vi "Read_Parse.vi"(0 "string in":string, 3 "Cluster in":T3) -> (1 "All Data":string, 4 "Motor DataString":string, 5 "DADES":T2, 6 "Acceleròmetre":T1, 7 "Giroscopi":T1, 9 "Magnetometre":T1, 10 "Cluster out":T3)   [LabVIEW 2018]
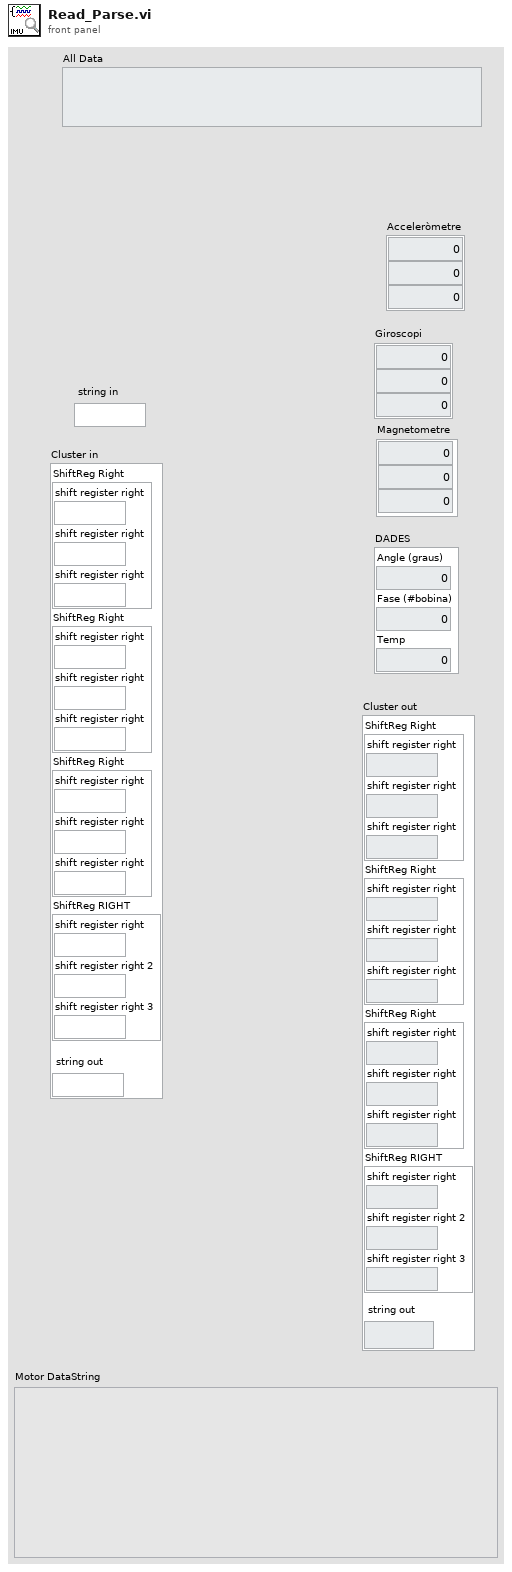
[diagram p1: front panel]
types:
  T1 = cluster{"Numeric":dbl, "Numeric":dbl, "Numeric":dbl}
  T2 = cluster{"Angle (graus)":dbl, "Fase (#bobina)":dbl, "Temp":dbl}
  T3 = cluster{"ShiftReg Right":cluster{"shift register right":string, "shift register right":string, "shift register right":string}, "ShiftReg Right":cluster{"shift register right":string, "shift register right":string, "shift register right":string}, "ShiftReg Right":cluster{"shift register right":string, "shift register right":string, "shift register right":string}, "ShiftReg RIGHT":cluster{"shift register right":string, "shift register right 2":string, "shift register right 3":string}, "\n string out":string}
  T4 = cluster{"shift register right":string, "shift register right":string, "shift register right":string}
  T5 = cluster{"shift register right":string, "shift register right 2":string, "shift register right 3":string}
  T6 = cluster{"ShiftReg Right":cluster{"shift register right":string, "shift register right":string, "shift register right":string}, "ShiftReg Right":cluster{"shift register right":string, "shift register right":string, "shift register right":string}, "ShiftReg Right":cluster{"shift register right":string, "shift register right":string, "shift register right":string}, "ShiftReg RIGHT":cluster{"shift register right":string, "shift register right 2":string, "shift register right 3":string}, "\n string in":string}
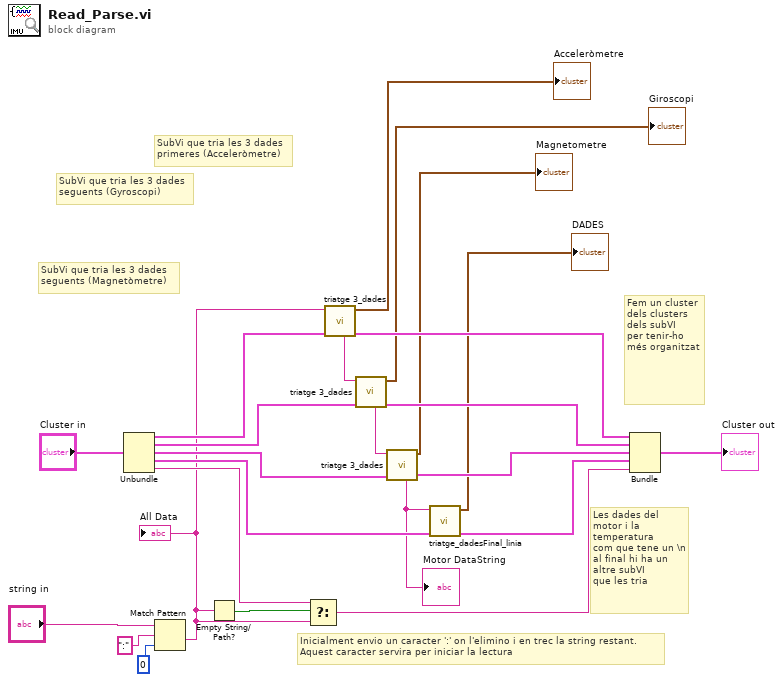
[diagram p0: block diagram]
diagram:
  # "SubVi que tria les 3 dades\nseguents (Magnetòmetre)"
  # "SubVi que tria les 3 dades\nseguents (Gyroscopi)"
  # "SubVi que tria les 3 dades\nprimeres (Acceleròmetre)"
  # "Inicialment envio un caracter ':' on l'elimino i en trec la string restant.\nAquest caracter servira per iniciar la lectura"
  # "Fem un cluster dels clusters dels subVI\nper tenir-ho més organitzat"
  # "Les dades del motor i la temperatura \ncom que tene un \\n al final hi ha un altre subVI\nque les tria"
  n1 = Unbundle("Cluster in") -> ("ShiftReg Right"=w18:T4, "ShiftReg Right"=w19:T4, "ShiftReg Right"=w20:T4, "ShiftReg RIGHT"=w21:T5, "string out"=w22:string)
  n2 = Match Pattern(string="string in", regular expression=":", offset (0)=0 ("t")) -> (after substring=w8:string)  [unwired: 3 out]
  "All Data" <- w8
  n3 = Empty String/Path?(string/path=w8) -> (empty?=w3:bool)
  n4 = Select(t=w22, s=w3, f=w8) -> (s? t:f=w15:string)
  n5 = call "triatge 3_dades.vi"("Cluster - Borderless"=w18, "DataIN"=w8) -> ("ShiftReg Right"=w11:T4, "Acceleròmetre"=→"Acceleròmetre":cluster{dbl, dbl, dbl}, "String Out"=w5:string)  [unwired: 7 in]
  n6 = call "triatge 3_dades.vi"("Cluster - Borderless"=w19, "DataIN"=w5) -> ("ShiftReg Right"=w12:T4, "Acceleròmetre"=→"Giroscopi":cluster{dbl, dbl, dbl}, "String Out"=w9:string)  [unwired: 7 in]
  n7 = call "triatge 3_dades.vi"("Cluster - Borderless"=w20, "DataIN"=w9) -> ("ShiftReg Right"=w13:T4, "Acceleròmetre"=→"Magnetometre":cluster{dbl, dbl, dbl}, "String Out"=w7:string)  [unwired: 7 in]
  "Motor DataString" <- w7
  n8 = call "triatge_dadesFinal_linia.vi"("ShiftReg LEFT"=w21, "String in"=w7) -> ("ShiftReg RIGHT"=w14:T5, "DADES"=→"DADES":T2)  [unwired: 8 in]
  n9 = Bundle("ShiftReg Right"=w11, "ShiftReg Right"=w12, "ShiftReg Right"=w13, "ShiftReg RIGHT"=w14, "string in"=w15) -> (→"Cluster out":T6)  [unwired: 1 in]
